vi "GenINI_Create_Constants.vi"(8 "error in":errorcluster, 9 "Data array":variant[](array[variant]), 10 "Terminal names":string[](array[string]), 11 "vi ref":refnum<vi>) -> (0 "error out":errorcluster, 3 "vi ref dup":refnum<vi>)   [LabVIEW 2009]
doc: "Create constants for named terminals on the owning block diagram for a given sub-vi."
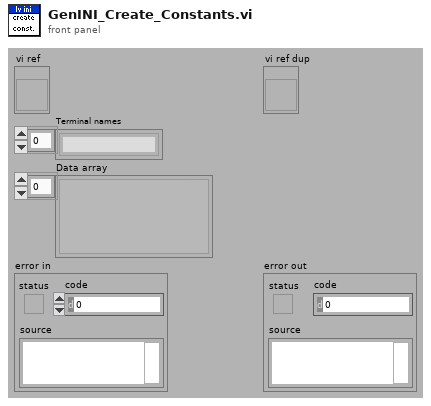
[diagram p1: front panel]
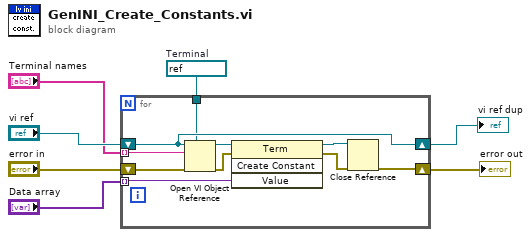
[diagram p0: block diagram]
diagram:
  w5 = refnum<vi> refnum  # Terminal
  n1 = for {
    tunnel: "Terminal names" -> [w17] mode=indexing
    shift-right: [w9] -> w7
    shift-left: "error in" -> [w14]
    tunnel: w5 -> [w12]
    tunnel: "Data array" -> [w11] mode=indexing
    shift-right: [w13] -> w6
    shift-left: "vi ref" -> [w13]
    n2 = Open VI Object Reference(7:w12, 8:w14, 10:w17, 11:w13) -> (0:w15:errorcluster, 3:w16:refnum<vi>)
    n3 = invoke class="Term" method="Create Constant"(reference=w16, error in=w15, "Value"=w11) -> (reference out=w10:refnum<vi>, error out=w8:errorcluster)  [unwired: 1 in, 2 out]
    n4 = Close Reference(reference=w10, error in (no error)=w8) -> (error out=w9:errorcluster)
  }
  "error out" <- w7
  "vi ref dup" <- w6
